vi "Insert In SubPanel.vi"(7 "SubPanel":refnum<vi>, 8 "error in (no error)":errorcluster, 11 "Interaction Splitter in":refnum<class "Interaction Splitter.lvclass">) -> (0 "error out":errorcluster, 3 "Interaction Splitter out":refnum<class "Interaction Splitter.lvclass">)   [LabVIEW 2021, in "Interaction Splitter.lvclass"]
doc: "Copyright 2018, Wiebe Walstra, wiebe@carya.nl."
uses:
  Interaction Splitter.lvclass
  Interaction Splitter.lvclass/Interaction Splitter.ctl
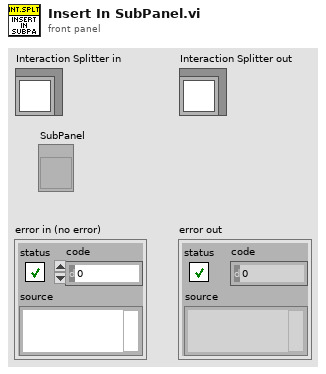
[diagram p1: front panel]
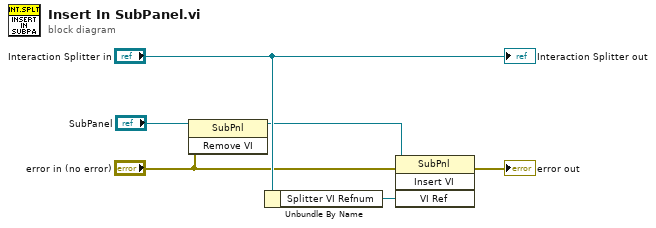
[diagram p0: block diagram]
diagram:
  n1 = invoke class="SubPnl" method="Remove VI"(reference="SubPanel", error in="error in (no error)") -> (reference out=w2:refnum<vi>)  [unwired: 1 in, 2 out]
  n2 = Unbundle By Name("Interaction Splitter in") -> ("Splitter VI Refnum"=w4:refnum<vi>)
  n3 = invoke class="SubPnl" method="Insert VI"(reference=w2, error in="error in (no error)", "VI Ref"=w4) -> (error out=→"error out":errorcluster)  [unwired: 1 in, 3 out]
  "Interaction Splitter out" <- "Interaction Splitter in"
